vi "Clear Finish Tasks.vi"(8 "error out":errorcluster, 9 "Music Paused":bool, 11 "Sounds In":T3(array[cluster]) {"Task ID" format="%.0x"}) -> (0 "error out":errorcluster, 3 "Sounds Out":T3(array[cluster]) {"Task ID" format="%.0x"})   [LabVIEW 2021, in "Sound Manager.lvlib"]
uses:
  Sound Manager.lvlib
  Typedefs/Sound Effects.ctl
  <vilib>/sound2/lvsound2.llb/Sound Output Task ID.ctl
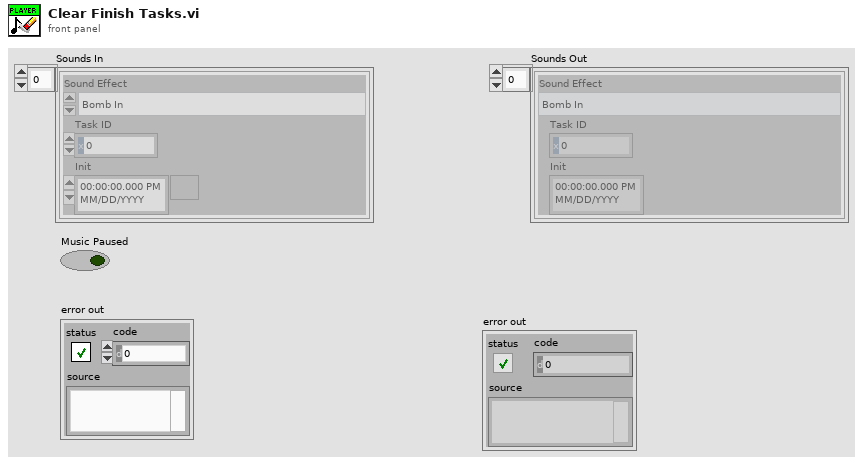
[diagram p1: front panel]
types:
  T1 = typedef "Sound Manager.lvlib/Sound Effects.ctl" = enum16{"Bomb In", "Bomb Out", "Bomb Touched", "Game Over", "Victory", "Eat", "10 Fruits", "Eat2", "Eat3", "Eat4", "MaxShield", "Shield", "10p", "Grape In", "Grape Out", "20p", "30p", "40p", "50p", "60p", "70p", "80p", "90p", "100p", "All shields cracked", "Mouse In", "Mouse Out", "Mouse Eaten", "Grape Eaten", "States Recover", "Broken Shield", "Bonus", "Happy Time", "explode", "Game over musica", "Back Music", "Shield Catch", "Evil lough", "Cricket In", "Cricket eaten", "Lets Go", "Jump1", "Jump2", "Jump3", "Unstoppable", "Troll Music", "winner"}
  T2 = typedef "Sound Output Task ID.ctl" = u32
  T3 = cluster{"Sound Effect":T1, "Task ID":T2, "Init":timestamp}[]
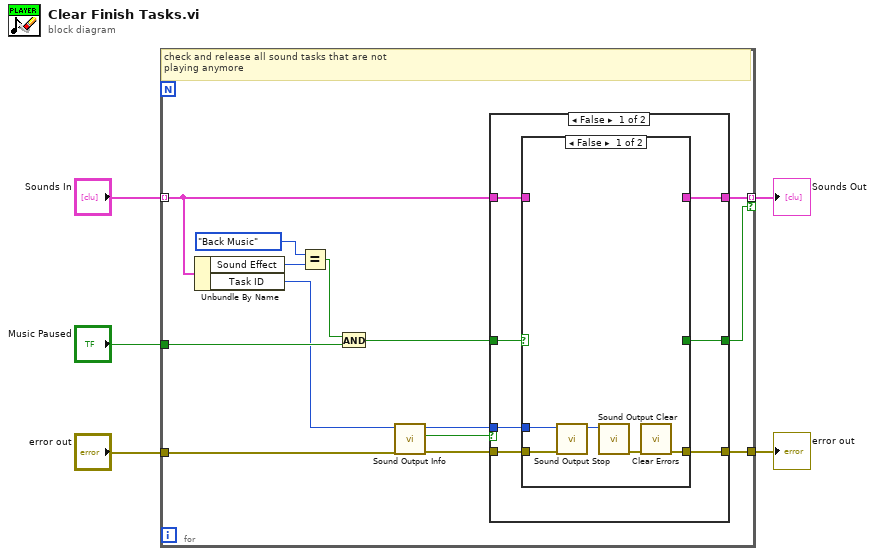
[diagram p0: block diagram]
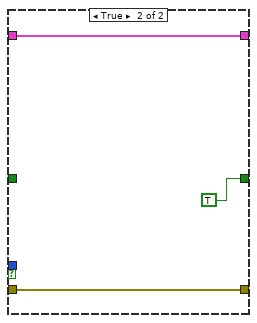
[diagram p3: hidden frame]
diagram:
  n1 = for {
    tunnel: "Sounds In" -> [w14] mode=indexing
    tunnel: [w16] -> w4 mode=indexing if=w15
    tunnel: "Music Paused" -> [w7]
    tunnel: "error out" -> [w9]
    tunnel: [w8] -> w1
    # "check and release all sound tasks that are not \nplaying anymore"
    n2 = Unbundle By Name(w14) -> ("Sound Effect"=w13:T1, "Task ID"=w6:T2)
    n3 = Equal?(x=Sound_Effects."Back Music" ("y"), y=w13) -> (x = y?=w11:bool)
    n4 = And(x=w11, y=w7) -> (x .and. y?=w10:bool)
    n5 = call <vilib>:"Sound Output Info.vi"("error in (no error)"=w9, "task ID"=w6) -> ("error out"=w18:errorcluster, "is playing?"=w19:bool, "task ID out"=w17:T2)  [unwired: 6 in, 1 out]
    n6 = case shown="False" w19 {
      tunnel: w18 -> [w26 w35]
      tunnel: w17 -> [w25 _]
      tunnel: [w21 w36] -> w16
      tunnel: [w23 TRUE] -> w15
      tunnel: w14 -> [w22 w36]
      tunnel: w10 -> [w24 _]
      tunnel: [w20 w35] -> w8
      frame False {
        n7 = case shown="False" w24 {
          selector: w24 -> [_ w34]
          tunnel: w26 -> [w29 w32]
          tunnel: w25 -> [w28 _]
          tunnel: [_ w34] -> w23
          tunnel: w22 -> [_ w33]
          tunnel: [_ w33] -> w21
          tunnel: [w27 w32] -> w20
          frame False {
            n8 = call <vilib>:"Sound Output Stop.vi"("error in (no error)"=w29, "task ID"=w28) -> ("task ID out"=w30:T2)  [unwired: 8 in, 1 out]
            n9 = call <vilib>:"Sound Output Clear.vi"("task ID"=w30) -> ("error out"=w31:errorcluster)  [unwired: 10 in]
            n10 = call <vilib>:"Clear Errors.vi"("error in (no error)"=w31) -> ("error out"=w27:errorcluster)  [unwired: 5 in, 1 out]
          }
          frame True {
            # "back music and paused, \ndo not clear"
          }
        }
      }
      frame True {
      }
    }
  }
  "Sounds Out" <- w4
  "error out" <- w1
